vi "Initialise DVR's.vi"(8 "error in (no error)":errorcluster, 11 "Type Counts":T2) -> (0 "error out":errorcluster, 3 "Data Value References":T1)   [LabVIEW 2021, in "Local Bus.lvclass"]
uses:
  Local Bus.lvclass
  Type Counts.ctl
  Data Value References.ctl
  <vilib>/TSA/Abstract Data Classes/Abs_Types/Type/Abs_Type.lvclass
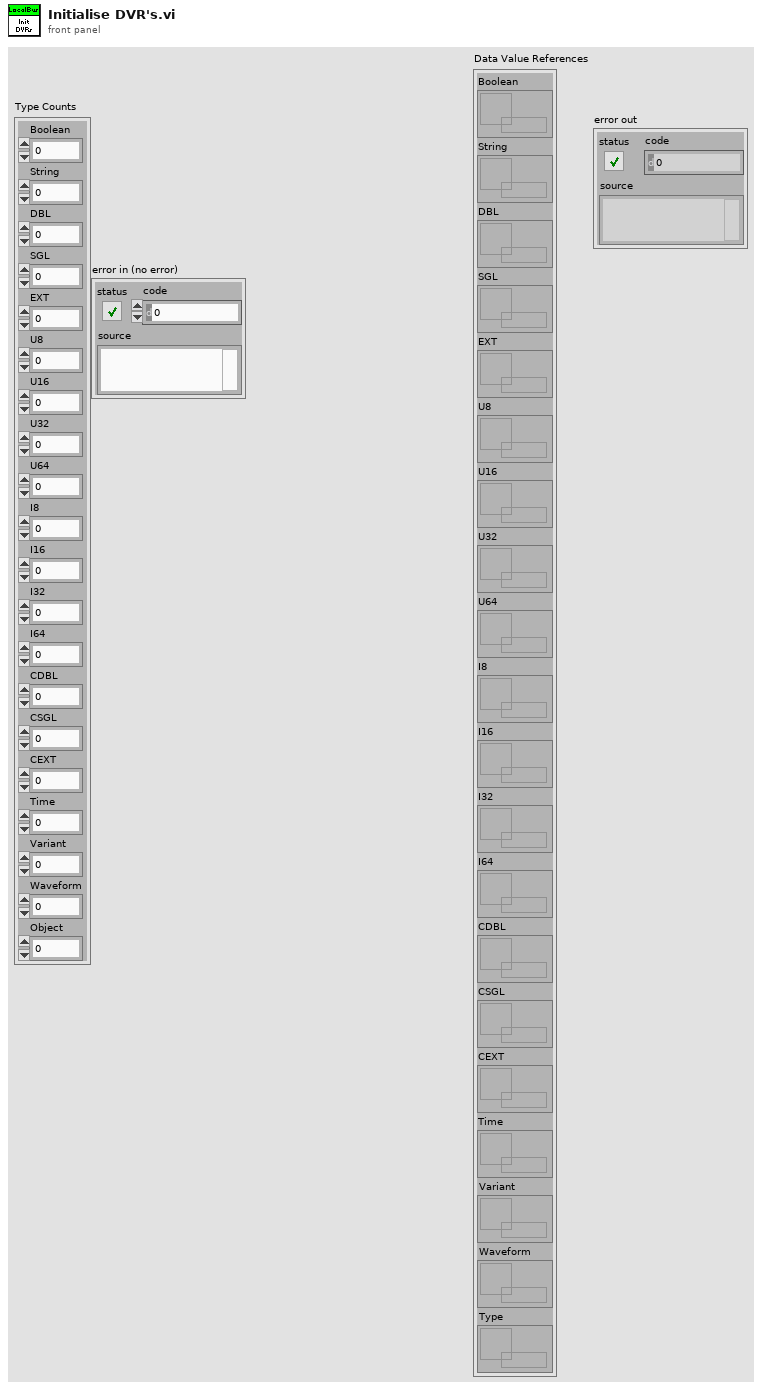
[diagram p1: front panel]
types:
  T1 = typedef "Local Bus.lvclass/Data Value References.ctl" = cluster{"Boolean":refnum<data-value>, "String":refnum<data-value>, "DBL":refnum<data-value>, "SGL":refnum<data-value>, "EXT":refnum<data-value>, "U8":refnum<data-value>, "U16":refnum<data-value>, "U32":refnum<data-value>, "U64":refnum<data-value>, "I8":refnum<data-value>, "I16":refnum<data-value>, "I32":refnum<data-value>, "I64":refnum<data-value>, "CDBL":refnum<data-value>, "CSGL":refnum<data-value>, "CEXT":refnum<data-value>, "Time":refnum<data-value>, "Variant":refnum<data-value>, "Waveform":refnum<data-value>, "Type":refnum<data-value>}
  T2 = typedef "Local Bus.lvclass/Type Counts.ctl" = cluster{"Boolean":i32, "String":i32, "DBL":i32, "SGL":i32, "EXT":i32, "U8":i32, "U16":i32, "U32":i32, "U64":i32, "I8":i32, "I16":i32, "I32":i32, "I64":i32, "CDBL":i32, "CSGL":i32, "CEXT":i32, "Time":i32, "Variant":i32, "Waveform":i32, "Object":i32}
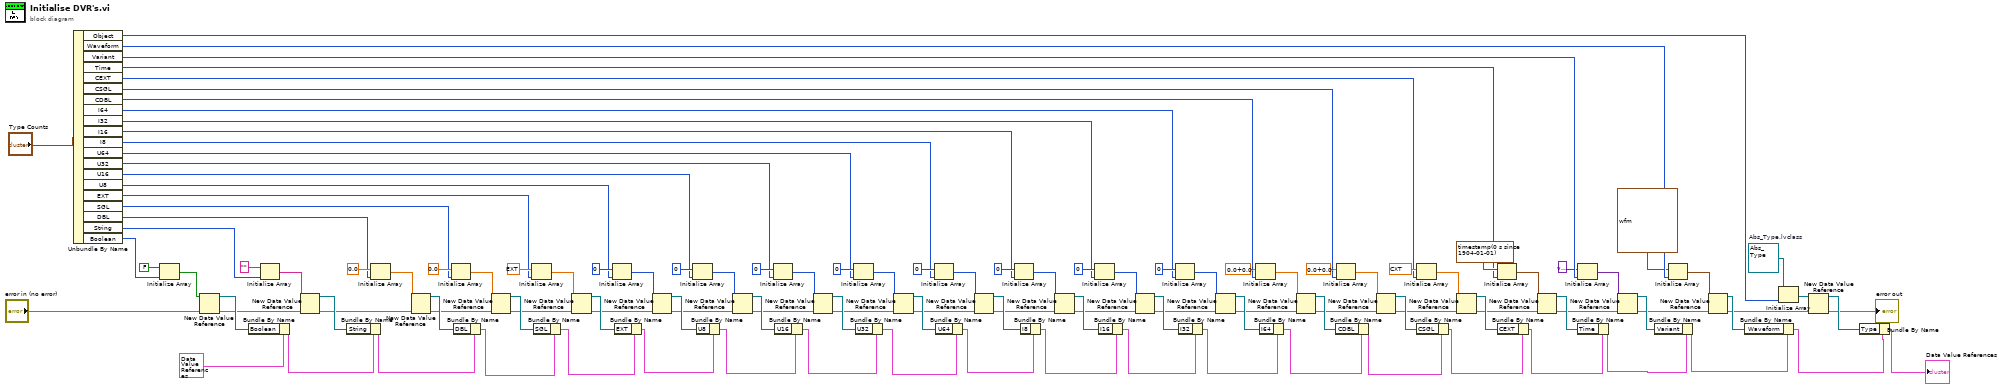
[diagram p0: block diagram]
diagram:
  w5 = refnum<class "Abs_Type.lvclass"> refnum  # Abs_Type.lvclass
  n1 = Unbundle By Name("Type Counts") -> ("Object"=w4:i32, "Waveform"=w27:i32, "Variant"=w28:i32, "Time"=w29:i32, "CEXT"=w30:i32, "CSGL"=w31:i32, "CDBL"=w32:i32, "I64"=w33:i32, "I32"=w34:i32, "I16"=w35:i32, "I8"=w71:i32, "U64"=w72:i32, "U32"=w73:i32, "U16"=w74:i32, "U8"=w75:i32, "EXT"=w76:i32, "SGL"=w77:i32, "DBL"=w106:i32, "String"=w112:i32, "Boolean"=w121:i32)
  n2 = Initialize Array(FALSE, w121) -> (w123:bool[])
  n3 = New Data Value Reference(data value=w123, error in="error in (no error)") -> (data value reference=w119:refnum<data-value>, error out=w115:errorcluster)
  n4 = Bundle By Name(cluster=T1 {"Boolean"=refnum, "String"=refnum, "DBL"=refnum, "SGL"=refnum, "EXT"=refnum, "U8"=refnum, "U16"=refnum, "U32"=refnum, "U64"=refnum, "I8"=refnum, "I16"=refnum, "I32"=refnum, "I64"=refnum, "CDBL"=refnum, "CSGL"=refnum, "CEXT"=refnum, "Time"=refnum, "Variant"=refnum, "Waveform"=refnum, "Type"=refnum} ("Data Value References"), "Boolean"=w119) -> (w117:T1)
  n5 = Initialize Array("", w112) -> (w116:string[])
  n6 = New Data Value Reference(data value=w116, error in=w115) -> (data value reference=w111:refnum<data-value>, error out=w108:errorcluster)
  n7 = Bundle By Name(cluster=w117, "String"=w111) -> (w105:T1)
  n8 = Initialize Array(0.0, w106) -> (w109:dbl[])
  n9 = New Data Value Reference(data value=w109, error in=w108) -> (data value reference=w110:refnum<data-value>, error out=w24:errorcluster)
  n10 = Initialize Array(sgl 0.0, w77) -> (w103:sgl[])
  n11 = Bundle By Name(cluster=w105, "DBL"=w110) -> (w83:T1)
  n12 = New Data Value Reference(data value=w103, error in=w24) -> (data value reference=w102:refnum<data-value>, error out=w23:errorcluster)
  n13 = Initialize Array(ext 0.0, w76) -> (w100:ext[])
  n14 = Bundle By Name(cluster=w83, "SGL"=w102) -> (w82:T1)
  n15 = New Data Value Reference(data value=w100, error in=w23) -> (data value reference=w101:refnum<data-value>, error out=w22:errorcluster)
  n16 = Initialize Array(u8 0, w75) -> (w97:u8[])
  n17 = Bundle By Name(cluster=w82, "EXT"=w101) -> (w81:T1)
  n18 = New Data Value Reference(data value=w97, error in=w22) -> (data value reference=w96:refnum<data-value>, error out=w21:errorcluster)
  n19 = Initialize Array(u16 0, w74) -> (w85:u16[])
  n20 = Bundle By Name(cluster=w81, "U8"=w96) -> (w80:T1)
  n21 = New Data Value Reference(data value=w85, error in=w21) -> (data value reference=w84:refnum<data-value>, error out=w20:errorcluster)
  n22 = Initialize Array(u32 0, w73) -> (w88:u32[])
  n23 = Bundle By Name(cluster=w80, "U16"=w84) -> (w79:T1)
  n24 = New Data Value Reference(data value=w88, error in=w20) -> (data value reference=w89:refnum<data-value>, error out=w19:errorcluster)
  n25 = Initialize Array(u64 0, w72) -> (w91:u64[])
  n26 = Bundle By Name(cluster=w79, "U32"=w89) -> (w78:T1)
  n27 = New Data Value Reference(data value=w91, error in=w19) -> (data value reference=w90:refnum<data-value>, error out=w18:errorcluster)
  n28 = Initialize Array(i8 0, w71) -> (w94:i8[])
  n29 = Bundle By Name(cluster=w78, "U64"=w90) -> (w47:T1)
  n30 = New Data Value Reference(data value=w94, error in=w18) -> (data value reference=w95:refnum<data-value>, error out=w17:errorcluster)
  n31 = Initialize Array(i16 0, w35) -> (w50:i16[])
  n32 = Bundle By Name(cluster=w47, "I8"=w95) -> (w46:T1)
  n33 = New Data Value Reference(data value=w50, error in=w17) -> (data value reference=w49:refnum<data-value>, error out=w16:errorcluster)
  n34 = Initialize Array(0, w34) -> (w52:i32[])
  n35 = Bundle By Name(cluster=w46, "I16"=w49) -> (w45:T1)
  n36 = New Data Value Reference(data value=w52, error in=w16) -> (data value reference=w53:refnum<data-value>, error out=w15:errorcluster)
  n37 = Initialize Array(i64 0, w33) -> (w55:i64[])
  n38 = Bundle By Name(cluster=w45, "I32"=w53) -> (w44:T1)
  n39 = New Data Value Reference(data value=w55, error in=w15) -> (data value reference=w54:refnum<data-value>, error out=w14:errorcluster)
  n40 = Initialize Array(cdb 0.0+0.0i, w32) -> (w58:cdb[])
  n41 = Bundle By Name(cluster=w44, "I64"=w54) -> (w43:T1)
  n42 = New Data Value Reference(data value=w58, error in=w14) -> (data value reference=w59:refnum<data-value>, error out=w13:errorcluster)
  n43 = Bundle By Name(cluster=w43, "CDBL"=w59) -> (w42:T1)
  n44 = Initialize Array(csg 0.0+0.0i, w31) -> (w69:csg[])
  n45 = New Data Value Reference(data value=w69, error in=w13) -> (data value reference=w70:refnum<data-value>, error out=w12:errorcluster)
  n46 = Bundle By Name(cluster=w42, "CSGL"=w70) -> (w41:T1)
  n47 = Initialize Array(cxt 0.0+0.0i, w30) -> (w66:cxt[])
  n48 = New Data Value Reference(data value=w66, error in=w12) -> (data value reference=w65:refnum<data-value>, error out=w11:errorcluster)
  n49 = Initialize Array(timestamp(0 s since 1904-01-01), w29) -> (w63:timestamp[])
  n50 = Bundle By Name(cluster=w41, "CEXT"=w65) -> (w40:T1)
  n51 = New Data Value Reference(data value=w63, error in=w11) -> (data value reference=w64:refnum<data-value>, error out=w10:errorcluster)
  n52 = Initialize Array(variant, w28) -> (w61:variant[])
  n53 = Bundle By Name(cluster=w40, "Time"=w64) -> (w39:T1)
  n54 = New Data Value Reference(data value=w61, error in=w10) -> (data value reference=w60:refnum<data-value>, error out=w9:errorcluster)
  n55 = Bundle By Name(cluster=w39, "Variant"=w60) -> (w37:T1)
  n56 = Initialize Array(waveform(dbl) {"t0"=timestamp(0 s since 1904-01-01), "dt"=1.0, "Y"=[]}, w27) -> (w38:waveform(dbl)[])
  n57 = New Data Value Reference(data value=w38, error in=w9) -> (data value reference=w36:refnum<data-value>, error out=w3:errorcluster)
  n58 = Bundle By Name(cluster=w37, "Waveform"=w36) -> (w8:T1)
  n59 = Initialize Array(w5, w4) -> (w6:refnum<class "Abs_Type.lvclass">[])
  n60 = New Data Value Reference(data value=w6, error in=w3) -> (data value reference=w7:refnum<data-value>, error out=→"error out":errorcluster)
  n61 = Bundle By Name(cluster=w8, "Type"=w7) -> (→"Data Value References":T1)
